vi "Configuration Keys.vi"(8 "error in":errorcluster, 11 "69X_79X in":refnum<class "7976A.lvclass">) -> (0 "error out":errorcluster, 2 "Required Keys":string[](array[string]), 3 "69X_79X out":refnum<class "7976A.lvclass">)   [LabVIEW 2019, in "7976A.lvlib" / "7976A.lvclass"]
doc: "Configuration Keys is a dynamic dispatch VI that reads a full inheritance chain's required key list.\n\nThis means each instrument must override this vi, and call the parent method . The end result is a comprehensive list of required keys that must be present in an instrument's config.ini file to correctly function."
uses:
  Library/7976A.lvclass
  builds/Instruments/PowerSupply.lvlibp/Library/PowerSupply.lvclass
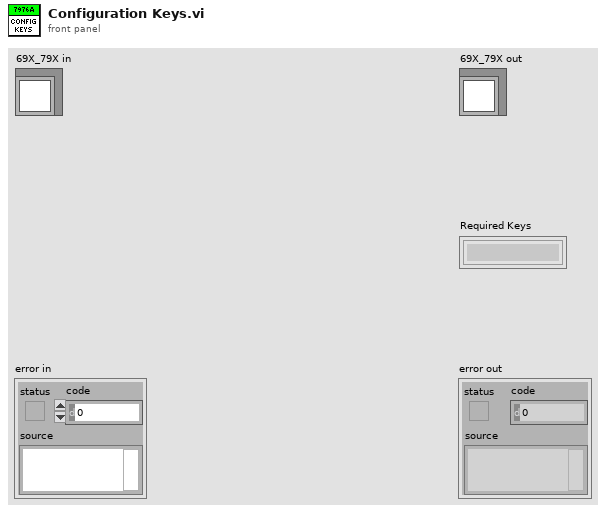
[diagram p1: front panel]
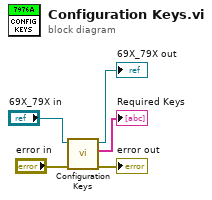
[diagram p0: block diagram]
diagram:
  n1 = call-parent "Configuration Keys.vi"("error in"="error in", "PowerSupply in"="69X_79X in") -> ("error out"=→"error out":errorcluster, "Required Keys"=→"Required Keys":string[], "PowerSupply out"=→"69X_79X out":refnum<class "7976A.lvclass">)  [unwired: 7 in]
